vi "_Pull Controls Value to DPs(VI).vi"(6 "sync DPs?(T)":bool=TRUE, 7 "VIRef(Caller VI)":refnum<vi>, 8 "error in (no error)":errorcluster, 9 "force update(F)":bool, 11 "SILAPI In":refnum<k1>) -> (0 "error out":errorcluster, 1 "Binded DPs":string[](array[string]), 3 "SILAPI Out":refnum<k1>)   [LabVIEW 2017, in "TagDB RefManager.lvlib"]
uses:
  TagDB RefManager.lvlib
  230c0da9-b6e4-44e0-8cb2-fe6bdec026ba.vi
  e135edd7-4a87-4b9d-b0c7-3b3f0cd11366.vi
  be640558-f0fc-44bb-96cd-108508b5fbdb.vi
  083faeab-0307-4387-9797-c882d96e285b.vi
  a032c900-6a26-4ad4-8296-bdd15205f1fc.vi
  024ec822-42c1-4cee-abf5-dbe2fbe4f70a.vi
  <userlib>/_NEVSTOP/TagDB/_Support/DataAccess/_NameCacher.vi
  <userlib>/_NEVSTOP/TagDB/_Support/Error/_[error50002]Invalid DataType.vi
  <userlib>/_NEVSTOP/TagDB/_Support/Error/_[error50000]Invalid DB REF.vi
  <userlib>/_NEVSTOP/TagDB/_Support/DataAccess/TagDB Ref to DVR.vi
  <userlib>/_NEVSTOP/TagDB/_Support/URL/TRIM-BOTH-SPACE.vi
  <userlib>/_NEVSTOP/TagDB/_Support/DataAccess/data-Write.vi
  <userlib>/_NEVSTOP/TagDB/_Support/DataAccess/_datatypeChecker.vi
  <userlib>/_NEVSTOP/TagDB/_Support/Error/_Build Error Cluster.vi
  <vilib>/Utility/Data Type/Get Type Information.vi
  <userlib>/_NEVSTOP/TagDB/TagDB.lvlib
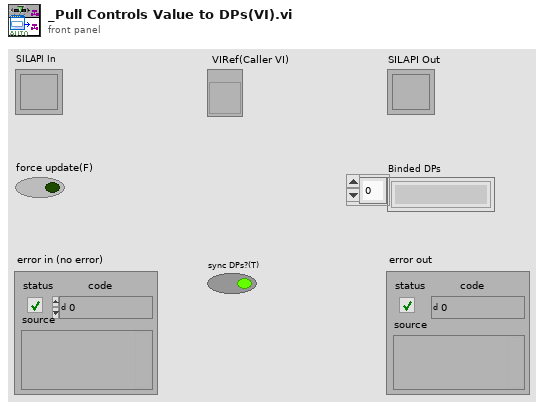
[diagram p1: front panel]
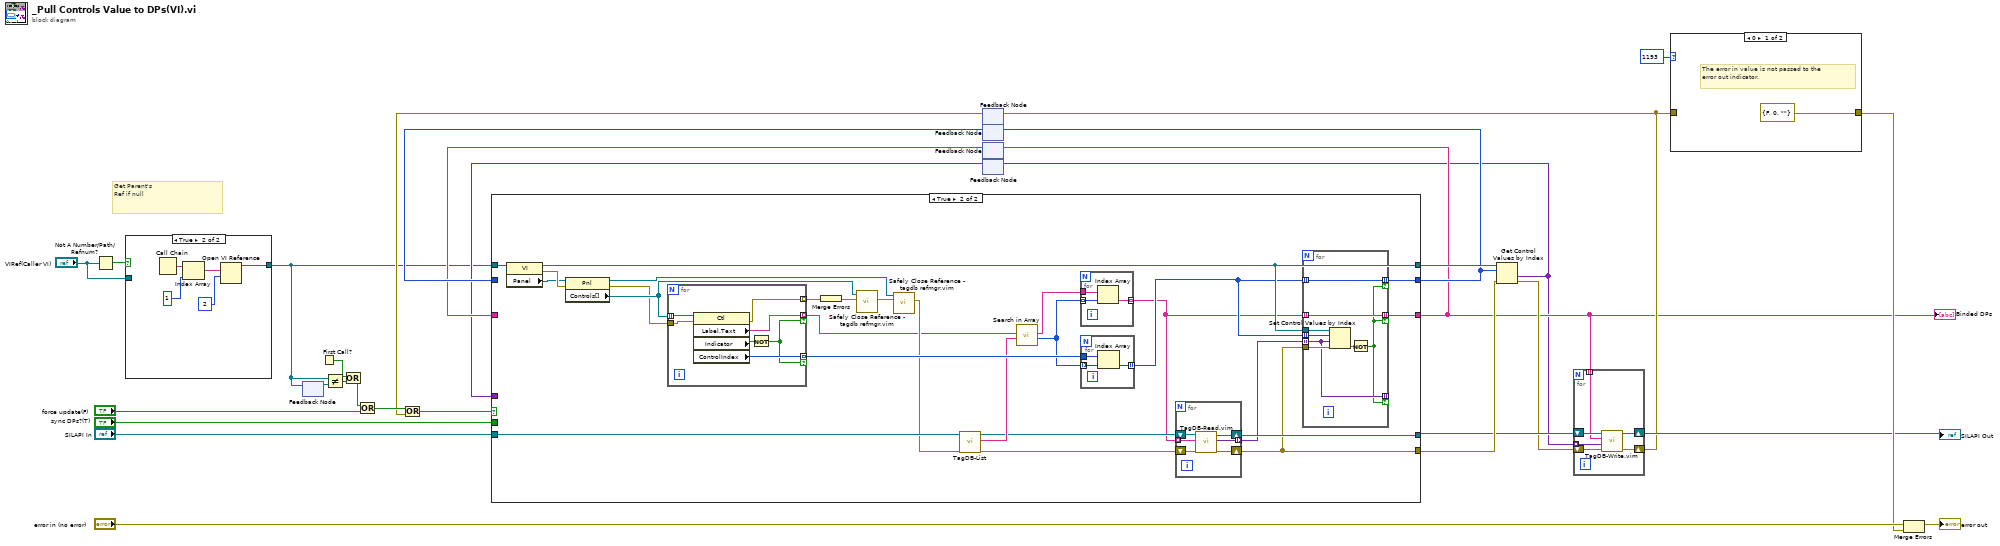
[diagram p0: block diagram]
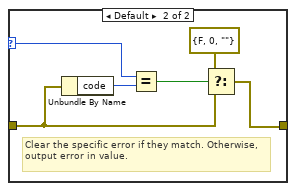
[diagram p3: hidden frame]
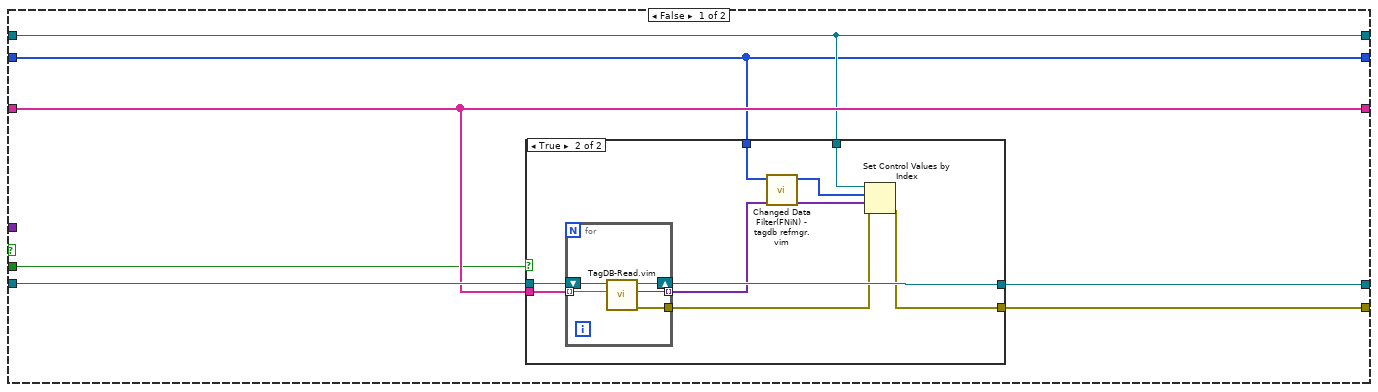
[diagram p4: hidden frame]
diagram:
  # "Get Parent's\nRef if null"
  n1 = Not A Number/Path/Refnum?(number/path/refnum="VIRef(Caller VI)") -> (NaN/Path/Refnum?=w7:bool)
  n2 = case shown="True" w7 {
    tunnel: [w30 w31] -> w1
    tunnel: "VIRef(Caller VI)" -> [w30 _]
    frame False {
    }
    frame True {
      n3 = Call Chain() -> (call chain=w35:string[])
      n4 = Index Array(array=w35, index=1 ("Index")) -> (element=w33:string)
      n5 = Open VI Reference(vi path=w33, options=2) -> (vi reference=w31:refnum<vi>)  [unwired: 4 in, 1 out]
    }
  }
  n6 = feedback #1() -> (w5:refnum<vi>)  [unwired: 1 in]
  n7 = feedback-in #1(w1) -> ()
  n8 = First Call?() -> (First Call?: T/F=w3:bool)
  n9 = Not Equal?(x=w1, y=w5) -> (x != y?=w4:bool)
  n10 = Or(x=w3, y=w4) -> (x .or. y?=w2:bool)
  n11 = Or(x=w2, y="force update(F)") -> (x .or. y?=w25:bool)
  n12 = feedback #2() -> (w17:errorcluster)  [unwired: 1 in]
  n13 = Or(x=w25, y=w17) -> (x .or. y?=w18:bool)
  n14 = feedback #3() -> (w26:i32[])  [unwired: 1 in]
  n15 = feedback #4() -> (w22:string[])  [unwired: 1 in]
  n16 = feedback #5() -> (w20:variant[])  [unwired: 1 in]
  n17 = case shown="True" w18 {
    tunnel: [w39 w74] -> w28
    tunnel: w1 -> [w39 w84]
    tunnel: [w37 w77] -> w27
    tunnel: w26 -> [w37 _]
    tunnel: [w41 w78] -> w10
    tunnel: w22 -> [w41 _]
    tunnel: "SILAPI In" -> [w42 w83]
    tunnel: [w38 w79] -> w15
    tunnel: w20 -> [_ _]
    tunnel: [w40 w81] -> w14
    tunnel: "sync DPs?(T)" -> [w36 _]
    frame False {
      n18 = case shown="True" w36 {
        tunnel: w42 -> [w43 w53]
        tunnel: w41 -> [_ w52]
        tunnel: [w43 w51] -> w40
        tunnel: w39 -> [_ w50]
        tunnel: [_ w48] -> w38
        tunnel: w37 -> [_ w45]
        frame False {
        }
        frame True {
          n19 = for {
            tunnel: w52 -> [w57] mode=indexing
            tunnel: [w55] -> w49
            tunnel: [w54] -> w47 mode=indexing
            shift-right: [w56] -> w51
            shift-left: w53 -> [w58]
            n20 = call "TagDB-Read.vim"("name"=w57, "TagDB"=w58) -> ("error out"=w55:errorcluster, "Value"=w54:variant, "TagDB(dup)"=w56:refnum<k1>)  [unwired: 4 in, 3 out]
          }
          n21 = call "Changed Data Filter(FNiN) - tagdb refmgr.vim"("checked data"=w47, "1"=w45) -> ("data"=w46:variant[], "1 out"=w44:i32[])  [unwired: 6 in, 2 out]
          n22 = Set Control Values by Index(0:w50, 1:w44, 2:w46, 3:w49) -> (11:w48:errorcluster)
        }
      }
    }
    frame True {
      n23 = property class="VI"(reference=w84) -> (reference out=w74:refnum<vi>, error out=w76:errorcluster, "Panel"=w75:refnum<vi>)  [unwired: 1 in]
      n24 = property class="Pnl"(reference=w75, error in=w76) -> (reference out=w68:refnum<vi>, error out=w65:errorcluster, "Controls[]"=w70:refnum<vi>[])
      n25 = for {
        tunnel: w70 -> [w103] mode=indexing
        tunnel: [w102] -> w62 mode=indexing if=w97
        tunnel: [w101] -> w73 mode=indexing if=w97
        tunnel: [w99] -> w71 mode=indexing
        tunnel: w65 -> [w98]
        n26 = property class="Ctl"(reference=w103, error in=w98) -> (error out=w99:errorcluster, "Label.Text"=w102:string, "Indicator"=w100:bool, "ControlIndex"=w101:i32)  [unwired: 1 out]
        n27 = Not(x=w100) -> (.not. x?=w97:bool)
      }
      n28 = Merge Errors(w71) -> (w69:errorcluster)
      n29 = call "Safely Close Reference - tagdb refmgr.vim"("error in (no error)"=w69, "Reference"=w70) -> ("error out"=w67:errorcluster)  [unwired: 9 in]
      n30 = call "Safely Close Reference - tagdb refmgr.vim"("error in (no error)"=w67, "Reference"=w68) -> ("error out"=w66:errorcluster)  [unwired: 9 in]
      n31 = call <userlib>:"TagDB-List.vi"("error in (no error)"=w66, "TagDB"=w83) -> ("error out"=w82:errorcluster, "names"=w64:string[], "TagDB(dup)"=w63:refnum<k1>)  [unwired: 6 in, 1 out]
      n32 = call "Search in Array.vi"("items to filter"=w64, "array"=w62) -> ("item Indexs"=w61:i32[], "array(dup)"=w59:string[])  [unwired: 4 in]
      n33 = for {
        tunnel: w61 -> [w87] mode=indexing
        tunnel: w59 -> [w86]
        tunnel: [w85] -> w60 mode=indexing
        n34 = Index Array(array=w86, index=w87) -> (element=w85:string)
      }
      n35 = for {
        tunnel: w61 -> [w90] mode=indexing
        tunnel: w73 -> [w89]
        tunnel: [w88] -> w72 mode=indexing
        n36 = Index Array(array=w89, index=w90) -> (element=w88:i32)
      }
      n37 = for {
        tunnel: [w94] -> w80 mode=indexing
        tunnel: w60 -> [w92] mode=indexing
        shift-right: [w93] -> w79
        shift-left: w82 -> [w96]
        shift-right: [w95] -> w81
        shift-left: w63 -> [w91]
        n38 = call "TagDB-Read.vim"("error in (no error)"=w96, "name"=w92, "TagDB"=w91) -> ("error out"=w93:errorcluster, "Value"=w94:variant, "TagDB(dup)"=w95:refnum<k1>)  [unwired: 3 in, 3 out]
      }
      n39 = for {
        tunnel: w74 -> [w111]
        tunnel: w72 -> [w110] mode=indexing
        tunnel: w80 -> [w106] mode=indexing
        tunnel: w79 -> [w109]
        tunnel: [w108] -> w78 mode=indexing if=w104
        tunnel: w60 -> [w108] mode=indexing
        tunnel: [w107] -> w77 mode=indexing if=w104
        tunnel: w72 -> [w107] mode=indexing
        tunnel: [w106] -> _ mode=indexing if=w104
        n40 = Set Control Values by Index(0:w111, 1:w110, 2:w106, 3:w109) -> (11:w105:errorcluster)
        n41 = Not(x=w105) -> (.not. x?=w104:bool)
      }
    }
  }
  "Binded DPs" <- w10
  n42 = feedback-in #3(w27) -> ()
  n43 = feedback-in #4(w10) -> ()
  n44 = Get Control Values by Index(0:w28, 1:w27, 3:w15) -> (10:w9:variant[], 11:w12:errorcluster)
  n45 = feedback-in #5(w9) -> ()
  n46 = for {
    tunnel: w9 -> [w113] mode=indexing
    shift-right: [w116] -> w13
    shift-left: w14 -> [w117]
    shift-right: [w114] -> w11
    shift-left: w12 -> [w115]
    tunnel: w10 -> [w112] mode=indexing
    n47 = call "TagDB-Write.vim"("error in (no error)"=w115, "Value"=w113, "tag"=w112, "TagDB"=w117) -> ("error out"=w114:errorcluster, "TagDB(dup)"=w116:refnum<k1>)  [unwired: 5 in, 1 out]
  }
  "SILAPI Out" <- w13
  n48 = feedback-in #2(w11) -> ()
  n49 = case shown="0" 1193 ("specific error code to clear (0: all)") {
    selector: 1193 ("specific error code to clear (0: all)") -> [_ w123]
    tunnel: w11 -> [_ w122]
    tunnel: [errorcluster {"status"=FALSE, "code"=0, "source"=""} ("error constant") w119] -> w19
    frame 0 {
      # "The error in value is not passed to the\nerror out indicator."
    }
    frame Default {
      # "Clear the specific error if they match. Otherwise, output error in value."
      n50 = Unbundle By Name(w122) -> ("code"=w124:i32)
      n51 = Equal?(x=w123, y=w124) -> (x = y?=w120:bool)
      n52 = Select(t=errorcluster {"status"=FALSE, "code"=0, "source"=""} ("error constant"), s=w120, f=w122) -> (s? t:f=w119:errorcluster)
    }
  }
  n53 = Merge Errors("error in (no error)", w19) -> (→"error out":errorcluster)
